vi "Response from Zoho creator.vi"(8 "error in":errorcluster, 11 "body":string) -> (0 "error out":errorcluster, 3 "decimated array":string[](array[string]))   [LabVIEW 2019, in "DataLogger.lvclass"]
uses:
  DataLogger.lvclass
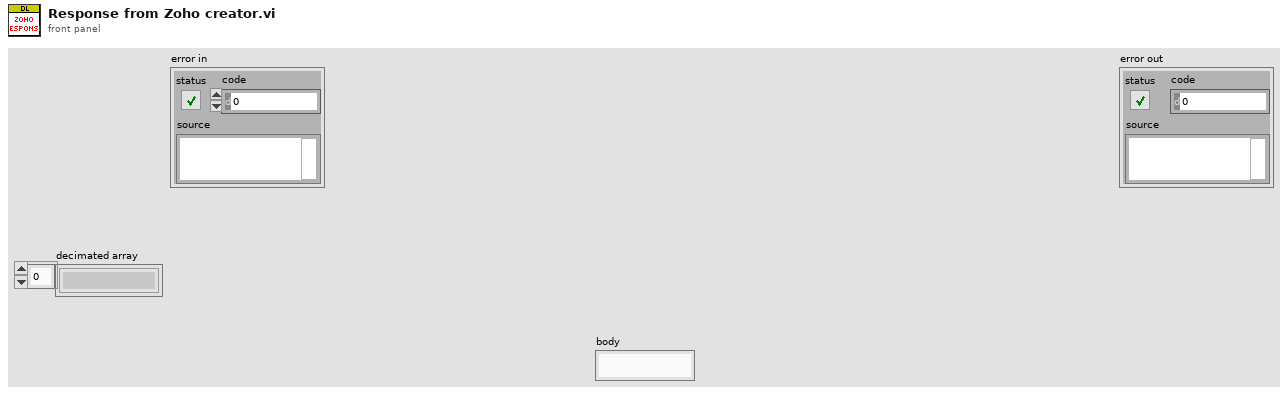
[diagram p1: front panel]
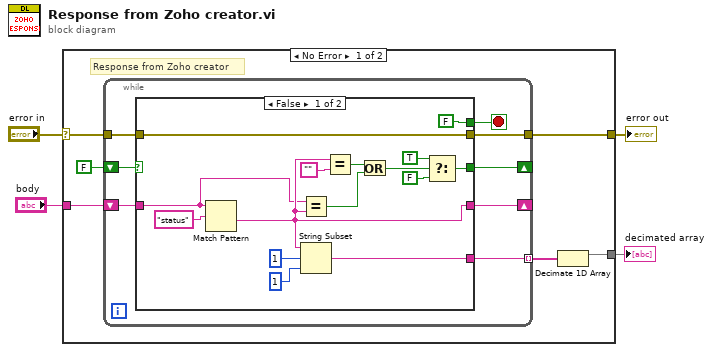
[diagram p0: block diagram]
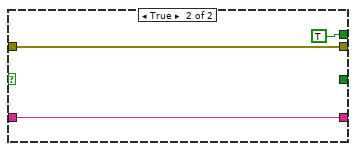
[diagram p2: hidden frame]
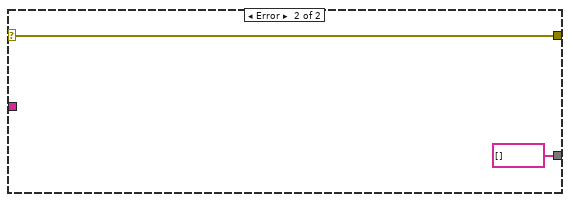
[diagram p3: hidden frame]
diagram:
  n1 = case shown="No Error" "error in" {
    selector: "error in" -> [w5 w38]
    tunnel: [w8 string[] []] -> w4
    tunnel: "body" -> [w7 _]
    tunnel: [w6 w38] -> w2
    frame No Error {
      # "Response from Zoho creator"
      n2 = while {
        shift-right: [w14] -> _
        shift-left: w7 -> [w16]
        shift-right: [w13] -> _
        shift-left: FALSE -> [w18]
        tunnel: [w15] -> w9 mode=indexing
        tunnel: w5 -> [w12]
        tunnel: [w11] -> w6
        stop <- w17 stop-if-true
        n3 = case shown="False" w18 {
          tunnel: [FALSE TRUE] -> w17
          tunnel: w16 -> [w23 w35]
          tunnel: [w29 _] -> w15
          tunnel: [w24 w35] -> w14
          tunnel: [w27 _] -> w13
          tunnel: w12 -> [w19 w34]
          tunnel: [w19 w34] -> w11
          frame False {
            n4 = Match Pattern(string=w23, regular expression="status") -> (after substring=w24:string)  [unwired: 1 in, 3 out]
            n5 = Equal?(x=w23, y=w24) -> (x = y?=w21:bool)
            n6 = String Subset(string=w24, offset (0)=1, length (rest)=1 ("length (rest)")) -> (substring=w29:string)
            n7 = Equal?(x=w24, y="") -> (x = y?=w20:bool)
            n8 = Or(x=w20, y=w21) -> (x .or. y?=w22:bool)
            n9 = Select(t=TRUE, s=w22, f=FALSE) -> (s? t:f=w27:bool)
          }
          frame True {
          }
        }
      }
      n10 = Decimate 1D Array(w9) -> (w8:string[])  [unwired: 1 out]
    }
    frame Error {
    }
  }
  "decimated array" <- w4
  "error out" <- w2
